vi "BL Source.vi"(8 "error in (no error)":errorcluster, 9 "settling time (s)":dbl=0.05 format="%#_6p", 10 "voltage level (V)":dbl=0.2 format="%#_6p", 11 "current limit range (A)":dbl=0.01 format="%#_6p") -> (0 "error out":errorcluster)   [LabVIEW 2019]
uses:
  <instrlib>/niDCPower/nidcpower.llb/niDCPower Source Mode.ctl
  <instrlib>/niDCPower/nidcpower.llb/niDCPower Wait For Event - Event.ctl
  <instrlib>/niDCPower/nidcpower.llb/niDCPower Output Function.ctl
  Globals.vi
panel:
  out "Channel Name":string="0"
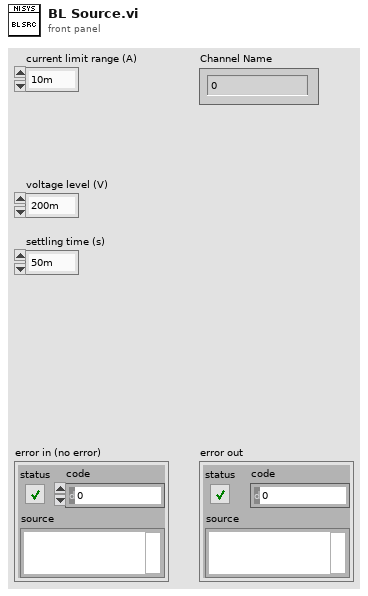
[diagram p1: front panel]
types:
  T1 = typedef "niDCPower Output Function.ctl" = i32
  T2 = typedef "niDCPower Wait For Event - Event.ctl" = i32
  T3 = typedef "niDCPower Source Mode.ctl" = i32
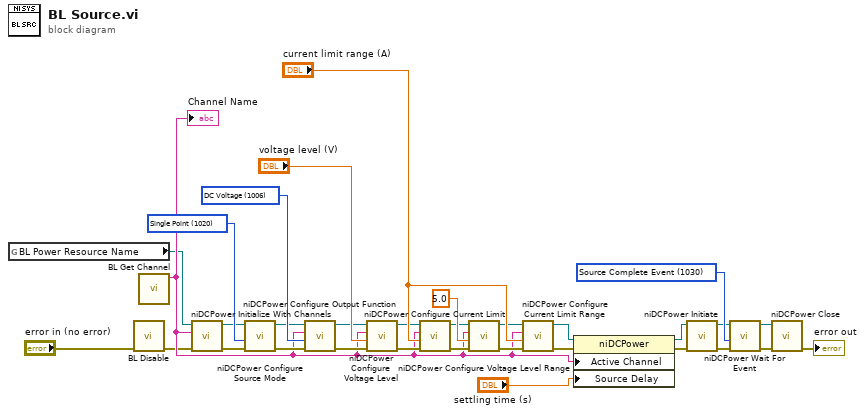
[diagram p0: block diagram]
diagram:
  w27 = T1 1006 items=["DC Voltage"=1006, "DC Current"=1007, "Pulse Voltage"=1049, "Pulse Current"=1050] ("output function")
  w24 = T2 1030 items=["Source Complete Event"=1030, "Measure Complete Event"=1031, "Sequence Iteration Complete Event"=1032, "Sequence Engine Done Event"=1033] ("event")
  w13 = T3 1020 items=["Single Point"=1020, "Sequence"=1021] ("source mode")
  n1 = global read "Globals.vi" "BL Power Resource Name"() -> (w1:refnum<k15>)
  n2 = call "BL Disable.vi"("error in (no error)"="error in (no error)") -> ("error out"=w2:errorcluster)  [unwired: 10 in]
  n3 = call "BL Get Channel.vi"() -> ("Channel Name"=w3:string)  [unwired: 10 in, 1 out]
  "Channel Name" <- w3
  n4 = call <instrlib>:"niDCPower Initialize With Channels.vi"("error in (no error)"=w2, "channels"=w3, "resource name"=w1) -> ("error out"=w9:errorcluster, "instrument handle out"=w10:refnum<k15>)  [unwired: 2 in, 5 out]
  n5 = call <instrlib>:"niDCPower Configure Source Mode.vi"("error in (no error)"=w9, "source mode"=w13, "instrument handle"=w10) -> ("error out"=w11:errorcluster, "instrument handle out"=w12:refnum<k15>)  [unwired: 7 out]
  n6 = call <instrlib>:"niDCPower Configure Output Function.vi"("error in (no error)"=w11, "output function"=w27, "channel name"=w3, "instrument handle"=w12) -> ("error out"=w26:errorcluster, "instrument handle out"=w25:refnum<k15>)  [unwired: 6 out]
  n7 = call <instrlib>:"niDCPower Configure Voltage Level.vi"("error in (no error)"=w26, "voltage level"="voltage level (V)", "channel name"=w3, "instrument handle"=w25) -> ("error out"=w8:errorcluster, "instrument handle out"=w7:refnum<k15>)  [unwired: 6 out]
  n8 = call <instrlib>:"niDCPower Configure Current Limit.vi"("error in (no error)"=w8, "current limit"="current limit range (A)", "channel name"=w3, "instrument handle"=w7) -> ("error out"=w14:errorcluster, "instrument handle out"=w15:refnum<k15>)  [unwired: 1 in, 5 out]
  n9 = call <instrlib>:"niDCPower Configure Voltage Level Range.vi"("error in (no error)"=w14, "voltage level range"=5.0, "channel name"=w3, "instrument handle"=w15) -> ("error out"=w16:errorcluster, "instrument handle out"=w17:refnum<k15>)  [unwired: 6 out]
  n10 = call <instrlib>:"niDCPower Configure Current Limit Range.vi"("error in (no error)"=w16, "current limit range"="current limit range (A)", "channel name"=w3, "instrument handle"=w17) -> ("error out"=w21:errorcluster, "instrument handle out"=w18:refnum<k15>)  [unwired: 6 out]
  n11 = property class="niDCPower"(reference=w18, error in=w21, "Active Channel"=w3, "Source Delay"="settling time (s)") -> (reference out=w19:refnum<k15>, error out=w20:errorcluster)
  n12 = call <instrlib>:"niDCPower Initiate.vi"("error in (no error)"=w20, "instrument handle"=w19) -> ("error out"=w23:errorcluster, "instrument handle out"=w22:refnum<k15>)  [unwired: 2 in, 6 out]
  n13 = call <instrlib>:"niDCPower Wait For Event.vi"("error in (no error)"=w23, "event"=w24, "instrument handle"=w22) -> ("error out"=w5:errorcluster, "instrument handle out"=w6:refnum<k15>)  [unwired: 1 in, 6 out]
  n14 = call <instrlib>:"niDCPower Close.vi"("error in (no error)"=w5, "instrument handle"=w6) -> ("error out"=→"error out":errorcluster)  [unwired: 9 out]
